vi "Result.Load Result Codes from XML File.vi"(8 "error in (no error)":errorcluster, 11 "Limit File Path":path) -> (0 "error out":errorcluster, 1 "Result Codes":T1[](array[typedef]), 2 "File Version":string, 3 "File Name":string, 4 "Limits in Variant":variant)   [LabVIEW 2018]
uses:
  Result.Result Code Item.ctl
  Result.Test Result Code File Data.ctl
panel:
  out "Test Name":string
  out "XML Version":string
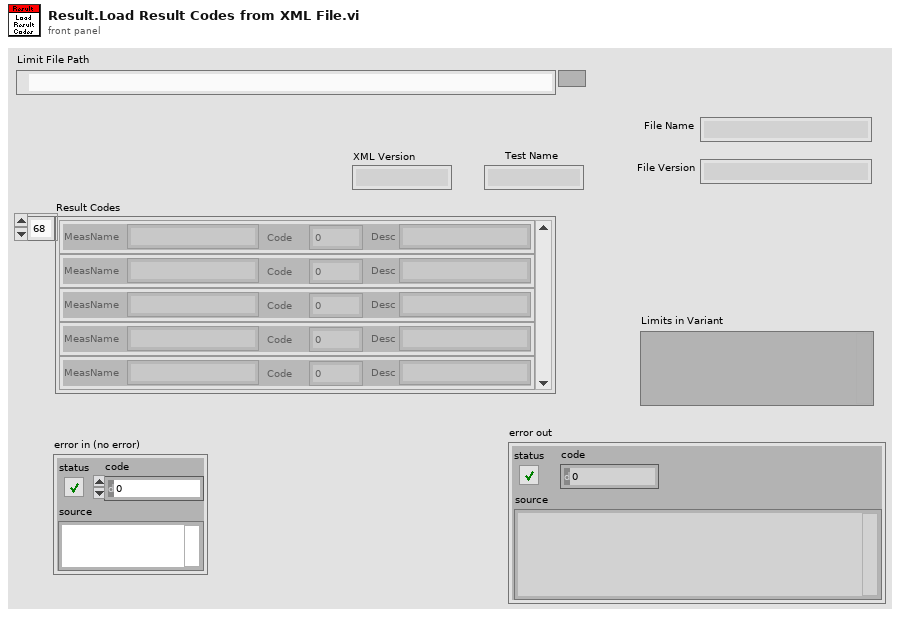
[diagram p1: front panel]
types:
  T1 = typedef "Result.Result Code Item.ctl" = cluster{"MeasName":string, "Code":i32, "Desc":string}
  T2 = typedef "Result.Test Result Code File Data.ctl" = cluster{"#attributes":cluster{"XMLFormatVer":string}, "TestName":string, "FileVersion":string, "CodePrefix":i32, "ResultCode":T1[]}
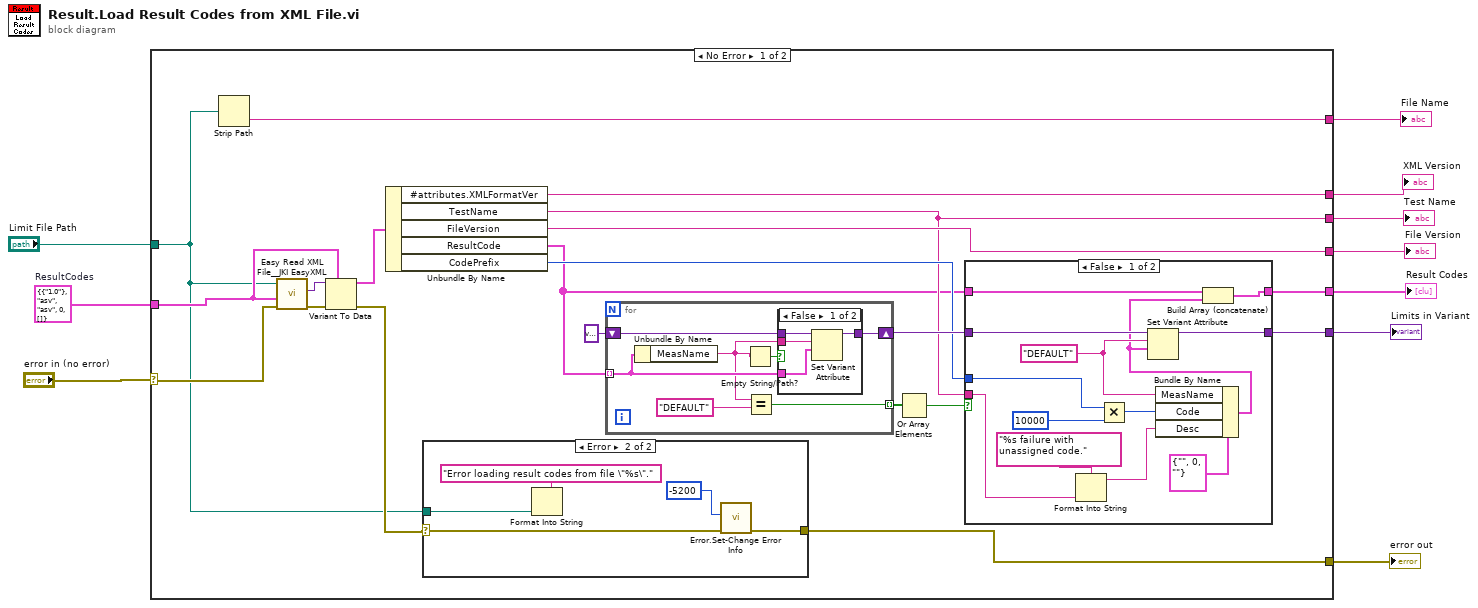
[diagram p0: block diagram]
diagram:
  w10 = T2 {"#attributes"={"XMLFormatVer"="1.0"}, "TestName"="asv", "FileVersion"="asv", "CodePrefix"=0, "ResultCode"=[]}  # ResultCodes
  n1 = case shown="No Error" "error in (no error)" {
    selector: "error in (no error)" -> [w22 w64]
    tunnel: w10 -> [w27 _]
    tunnel: [w26 _] -> w9
    tunnel: [w14 _] -> w8
    tunnel: [w25 _] -> w7
    tunnel: "Limit File Path" -> [w19 _]
    tunnel: [w24 _] -> w5
    tunnel: [w12 _] -> w4
    tunnel: [w16 _] -> w3
    tunnel: [w20 w64] -> w1
    frame No Error {
      n2 = Strip Path(path=w19) -> (name=w24:string)  [unwired: 1 out]
      n3 = call <vilib>:"Easy Read XML File__JKI EasyXML.vi"("error in (no error)"=w22, "LabVIEW Data (Type)"=w27, "XML File Path"=w19) -> ("error out"=w30:errorcluster, "LabVIEW Data"=w29:variant)  [unwired: 6 in, 1 out]
      n4 = Variant To Data(error in=w30, type=w27, Variant=w29) -> (data=w28:T2, error out=w21:errorcluster)
      n5 = Unbundle By Name(w28) -> ("#attributes.XMLFormatVer"=w26:string, "TestName"=w14:string, "FileVersion"=w25:string, "ResultCode"=w11:T1[], "CodePrefix"=w15:i32)
      n6 = case shown="Error" w21 {
        selector: w21 -> [w46 w51]
        tunnel: [w46 w49] -> w20
        tunnel: w19 -> [_ w47]
        frame No Error {
        }
        frame Error {
          n7 = Format Into String(format string="Error loading result codes from file \"%s\".", w47) -> ()  [unwired: 2 in, 2 out]
          n8 = call "Error.Set-Change Error Info.vi"("error in"=w51, "Cust Code(0 = no change)"=-5200 ("code")) -> ("error out"=w49:errorcluster)  [unwired: 9 in]
        }
      }
      n9 = for {
        tunnel: w11 -> [w56] mode=indexing
        shift-right: [w57] -> w17
        shift-left: variant ("Limits in Variant") -> [w58]
        tunnel: [w54] -> w18 mode=indexing
        n10 = Unbundle By Name(w56) -> ("MeasName"=w52:string)
        n11 = Empty String/Path?(string/path=w52) -> (empty?=w53:bool)
        n12 = Equal?(x=w52, y="DEFAULT") -> (x = y?=w54:bool)
        n13 = case shown="False" w53 {
          tunnel: w58 -> [w62 w63]
          tunnel: [w61 w63] -> w57
          tunnel: w56 -> [w60 _]
          tunnel: w52 -> [w59 _]
          frame False {
            n14 = Set Variant Attribute(Variant=w62, name=w59, value=w60) -> (Variant out=w61:variant)  [unwired: 1 in, 2 out]
          }
          frame True {
          }
        }
      }
      n15 = Or Array Elements(Boolean array=w18) -> (logical OR=w13:bool)
      n16 = case shown="False" w13 {
        tunnel: w17 -> [w43 w45]
        tunnel: [w42 w45] -> w16
        tunnel: w15 -> [w34 _]
        tunnel: w14 -> [w36 _]
        tunnel: [w33 w44] -> w12
        tunnel: w11 -> [w32 w44]
        frame False {
          w38 = "DEFAULT" ("y")
          n17 = Format Into String(format string="%s failure with unassigned code." ("y"), w36) -> (resulting string=w35:string)  [unwired: 2 in, 1 out]
          n18 = Multiply(x=w34, y=10000) -> (x*y=w39:i32)
          n19 = Bundle By Name(cluster=T1 {"MeasName"="", "Code"=0, "Desc"=""} ("Result.Result Code Item"), "MeasName"=w38, "Code"=w39, "Desc"=w35) -> (w31:T1)
          n20 = Set Variant Attribute(Variant=w43, name=w38, value=w31) -> (Variant out=w42:variant)  [unwired: 1 in, 2 out]
          n21 = Build Array (concatenate)(w32, w31) -> (w33:T1[])
        }
        frame True {
        }
      }
    }
    frame Error {
    }
  }
  "Result Codes" <- w4
  "XML Version" <- w9
  "File Name" <- w5
  "File Version" <- w7
  "Test Name" <- w8
  "Limits in Variant" <- w3
  "error out" <- w1
